vi "deregister.vi"(0 "HGF_DSCMonitor":refnum<class "HGF_DSCMonitor.lvclass">, 1 "SV":string, 2 "HGF_NetworkVisitor":refnum<class "HGF_NetworkVisitor.lvclass">, 3 "HGF_TriggeredEvent":refnum<class "HGF_TriggeredEvent.lvclass">, 4 "Rem SV/Visitor from List":bool, 5 "error in (no error)":errorcluster) -> (14 "HGF_DSCMonitor":refnum<class "HGF_DSCMonitor.lvclass">, 19 "error out":errorcluster)   [LabVIEW 2012, in "HGF_DSC.lvlib" / "HGF_DSCMonitor.lvclass"]
uses:
  HGF_DSCMonitor.lvclass
  HGF_BaseClasses/HGF_TriggeredEvent/HGF_TriggeredEvent.lvclass
  HGF_BaseClasses/HGF_NetworkVisitor/HGF_NetworkVisitor.lvclass
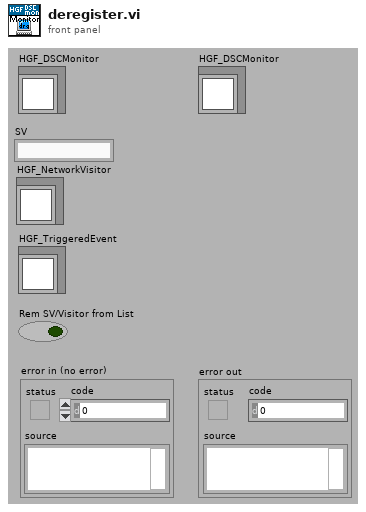
[diagram p1: front panel]
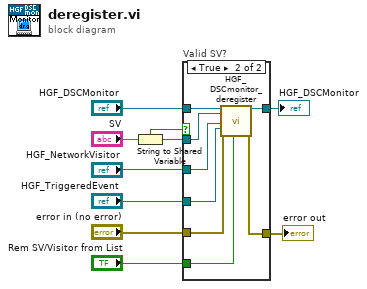
[diagram p0: block diagram]
diagram:
  n1 = String to Shared Variable(0:"SV") -> (1:w1:bool, 2:w2:refnum<k21>)
  n2 = case "Valid SV?" shown="True" w1 {
    tunnel: "HGF_DSCMonitor" -> [w12 w20]
    tunnel: [w12 w19] -> w9
    tunnel: "HGF_NetworkVisitor" -> [_ w18]
    tunnel: "HGF_TriggeredEvent" -> [_ w17]
    tunnel: "error in (no error)" -> [w11 w16]
    tunnel: "Rem SV/Visitor from List" -> [_ w15]
    tunnel: [w11 w14] -> w4
    tunnel: w2 -> [_ w13]
    frame False {
    }
    frame True {
      n3 = call "HGF_DSCmonitor_deregister.vi"("HGF_DSCMonitor in"=w20, "SV"=w13, "HGF_NetworkVisitor"=w18, "HGF_TriggeredEvent"=w17, "error in (no error)"=w16, "Rem SV/Visitor from List"=w15) -> ("HGF_DSCMonitor out"=w19:refnum<class "HGF_DSCMonitor.lvclass">, "error out"=w14:errorcluster)  [unwired: 12 in]
    }
  }
  "error out" <- w4
  "HGF_DSCMonitor" <- w9
